vi "get_file.vi"() -> ()   [LabVIEW 2017]
uses:
  <vilib>/rvi/interface/RandomDataEmulation/nirviRandomDataOpen.vi
  <vilib>/rvi/interface/common/niFpgaCacheSessionInfoDynamic.vi
  <vilib>/Utility/error.llb/Error Cluster From Error Code.vi
  <vilib>/rvi/errors/niLvFpgaAdjustHostInterfaceError.vi
  <vilib>/rvi/interface/nirviOpenFPGA/nirviOpenFPGA.xnode
  filter.vi
  <vilib>/rvi/interface/nirviMethod/nirviMethod.xnode
  <vilib>/rvi/errors/niLvFpgaMergeErrorWithErrorCode.vi
  <vilib>/FPGAPlugInAG/Dynamic/niLvFpga_ReadFifo_Dynamic.vi
  <vilib>/FPGAPlugInAG/Dynamic/niLvFpga_WriteFifo_Dynamic.vi
panel:
  out "Numeric":dbl
  out "Current index":dbl
  out "Total number of index":dbl
  out "downstream chart":sgl[](graph)
  in  "path":path=path "C:/Users/jte01/Music/John_Wesley_FILEN.wav"
  out "upstream chart":dbl(graph)
  out "dt":dbl
  out "Wav file Amplitude graph":dbl[](graph)
  out "t0":timestamp
  out "Waveform Graph":waveform(dbl)(graph)
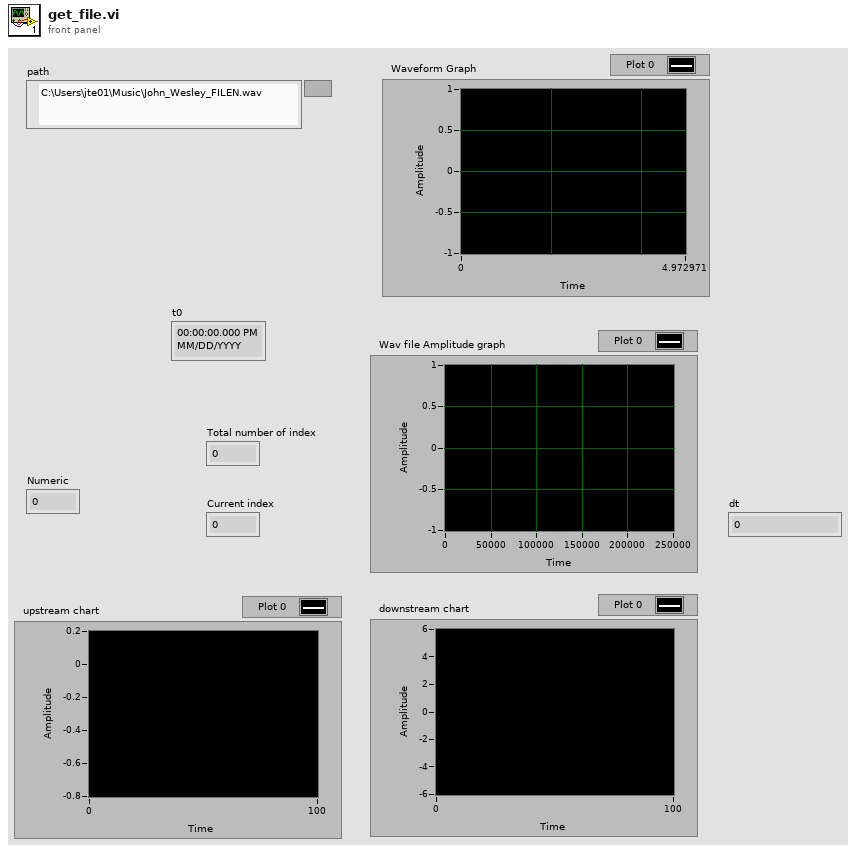
[diagram p1: front panel]
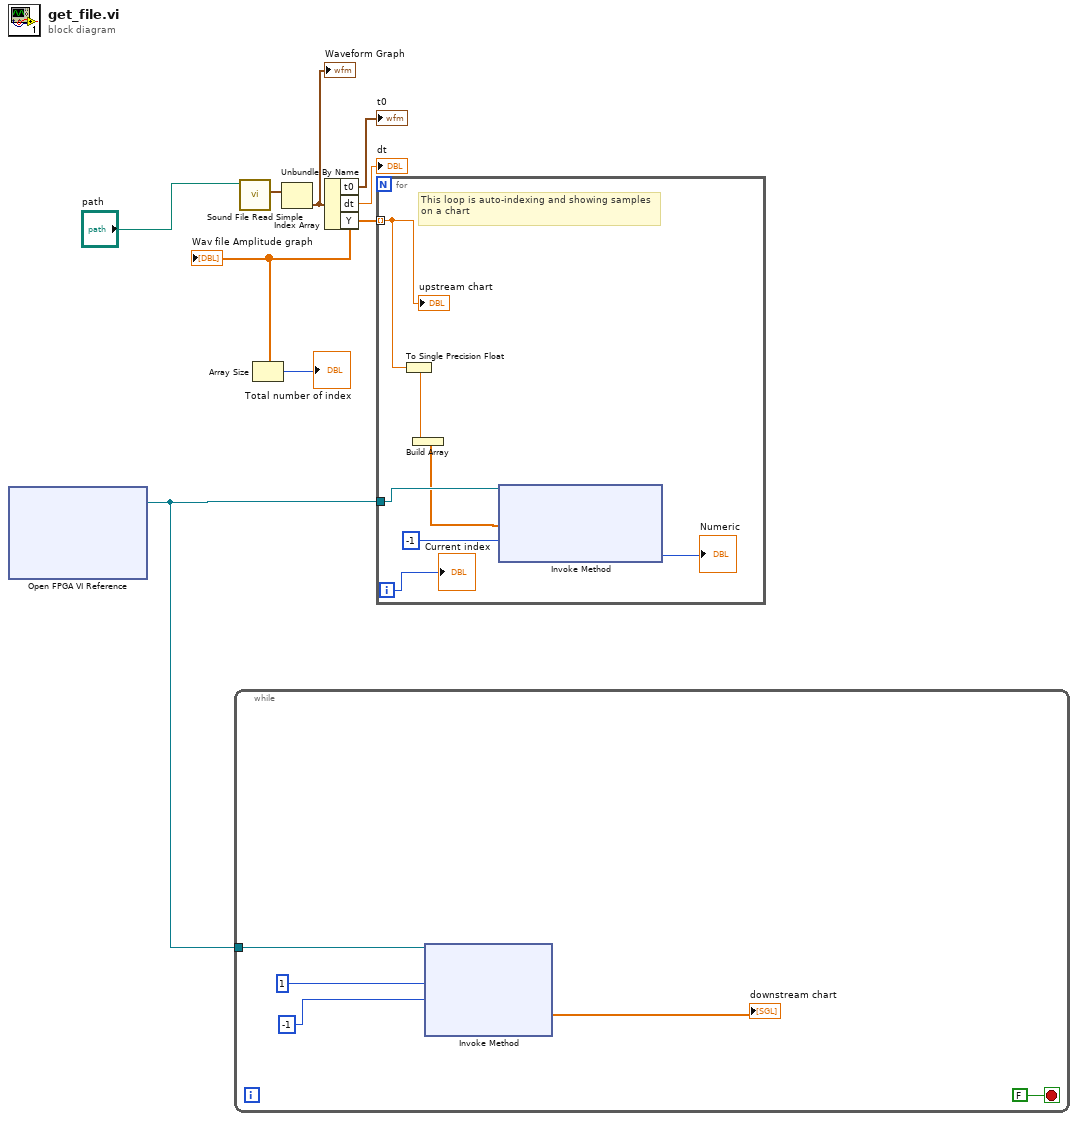
[diagram p0: block diagram]
diagram:
  n1 = xnode "Open FPGA VI Reference"() -> ("FPGA VI Reference Out"=w3:refnum<k20>)  [unwired: 2 in, 1 out]
  n2 = while {
    tunnel: w3 -> [w12]
    stop <- FALSE stop-if-true
    n3 = xnode "Invoke Method"("FPGA VI Reference In"=w12, "Number of Elements"=1, "Timeout (ms)"=-1) -> ("Data"=→"downstream chart":sgl[])  [unwired: 1 in, 3 out]
  }
  n4 = call <vilib>:"Sound File Read Simple.vi"("path"="path") -> ("data"=w4:waveform(dbl)[])  [unwired: 7 in, 3 out]
  n5 = Index Array(array=w4) -> (element=w8:waveform(dbl))  [unwired: 1 in]
  "Waveform Graph" <- w8
  n6 = Unbundle By Name(w8) -> ("t0"=→"t0":timestamp, "dt"=→"dt":dbl, "Y"=w2:dbl[])
  "Wav file Amplitude graph" <- w2
  n7 = Array Size(array=w2) -> (size(s)=→"Total number of index":i32)
  n8 = for {
    tunnel: w2 -> [w18] mode=indexing
    tunnel: w3 -> [w20]
    i -> [w15]
    # "This loop is auto-indexing and showing samples on a chart"
    n9 = To Single Precision Float(number=w18) -> (single precision float=w17:sgl)
    n10 = Build Array(w17) -> (w16:sgl[])
    n11 = xnode "Invoke Method"("FPGA VI Reference In"=w20, "Data"=w16, "Timeout (ms)"=-1) -> ("Empty Elements Remaining"=→"Numeric":u32)  [unwired: 1 in, 2 out]
    "upstream chart" <- w18
    "Current index" <- w15
  }
